vi "ziListDevices.vi"(4 "Error In":errorcluster, 7 "Handle In":T1 {"Handle" format="0x%08x"; "Conn" format="0x%08x"}) -> (0 "Error Out":errorcluster, 2 "Devices":cluster{"Nodes":string, i32}[](array[cluster]), 3 "Handle Out":T1 {"Handle" format="0x%08x"; "Conn" format="0x%08x"})   [LabVIEW 2016, in "Zurich Instruments LabOne.lvlib"]
doc: "Returns a list of ZI Instruments that are available in the connected Data Server."
uses:
  Zurich Instruments LabOne.lvlib
  ziTypeHandle.ctl
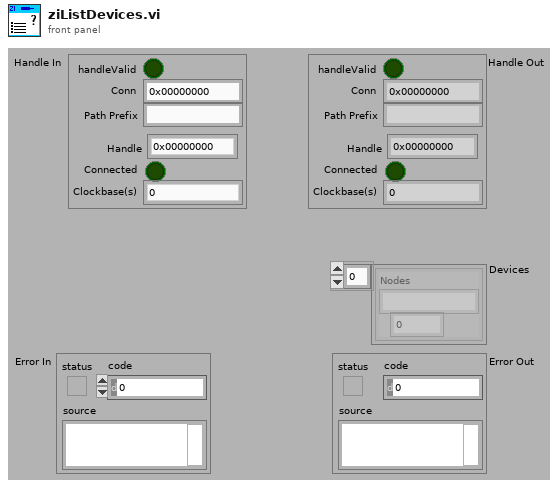
[diagram p1: front panel]
types:
  T1 = typedef "Zurich Instruments LabOne.lvlib/ziTypeHandle.ctl" = cluster{"handleValid":bool, "Conn":u64, "Path Prefix":string, "Handle":u64, "Connected":bool, "Clockbase(s)":dbl}
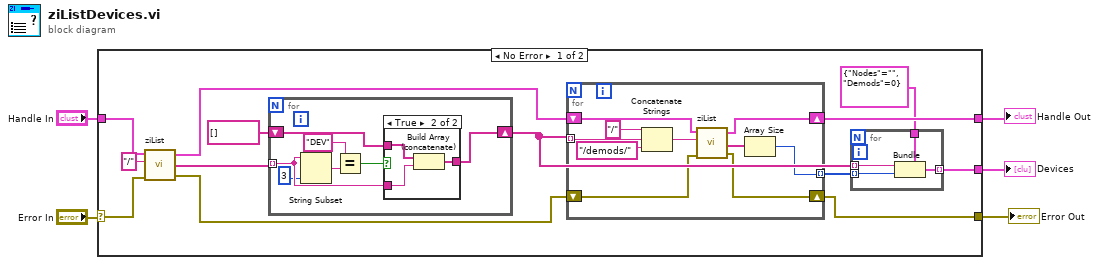
[diagram p0: block diagram]
diagram:
  n1 = case shown="No Error" "Error In" {
    selector: "Error In" -> [w6 w45]
    tunnel: "Handle In" -> [w17 w44]
    tunnel: [w15 w44] -> w4
    tunnel: [w14 w45] -> w3
    tunnel: [w11 _] -> w2
    frame No Error {
      n2 = call "ziList.vi"("Error In"=w6, "Path (\"\")"="/" ("Path (\"\")"), "Handle In"=w17) -> ("Error Out"=w10:errorcluster, "Nodes"=w16:string[], "Handle Out"=w9:T1)  [unwired: 1 out]
      n3 = for {
        tunnel: w16 -> [w36] mode=indexing
        shift-right: [w34] -> w13
        shift-left: string[] [] -> [w35]
        n4 = String Subset(string=w36, length (rest)=3 ("length (rest)")) -> (substring=w39:string)  [unwired: 1 out]
        n5 = Equal?(x="DEV", y=w39) -> (x = y?=w37:bool)
        n6 = case shown="True" w37 {
          tunnel: w36 -> [_ w42]
          tunnel: w35 -> [w40 w43]
          tunnel: [w40 w41] -> w34
          frame False {
          }
          frame True {
            n7 = Build Array (concatenate)(w43, w42) -> (w41:string[])
          }
        }
      }
      n8 = for {
        tunnel: w13 -> [w31] mode=indexing
        shift-right: [w25] -> w15
        shift-left: w9 -> [w28]
        shift-right: [w27] -> w14
        shift-left: w10 -> [w26]
        tunnel: [w23] -> w12 mode=indexing
        n9 = Concatenate Strings("/" ("x"), w31, "/demods/" ("x")) -> (w29:string)
        n10 = call "ziList.vi"("Error In"=w26, "Path (\"\")"=w29, "Handle In"=w28) -> ("Error Out"=w27:errorcluster, "Nodes"=w24:string[], "Handle Out"=w25:T1)  [unwired: 1 out]
        n11 = Array Size(array=w24) -> (size(s)=w23:i32)
      }
      n12 = for {
        tunnel: w13 -> [w22] mode=indexing
        tunnel: w12 -> [w21] mode=indexing
        tunnel: [w20] -> w11 mode=indexing
        tunnel: cluster{"Nodes":string, "Demods":i32} {"Nodes"="", "Demods"=0} ("cluster") -> [w19]
        n13 = Bundle(cluster=w19, "Nodes"=w22, "Demods"=w21) -> (w20:cluster{"Nodes":string, "Demods":i32})
      }
    }
    frame Error {
    }
  }
  "Handle Out" <- w4
  "Error Out" <- w3
  "Devices" <- w2
